vi "_getNbOfElements.vi"(11 "VariantBuffer in":refnum<class "VariantBuffer.lvclass">) -> (2 "nbElements":i32)   [LabVIEW 2013, in "CircularBuffer.lvlib" / "VariantBuffer.lvclass"]
uses:
  VariantBuffer.lvclass
  VariantBuffer.lvclass/VariantBuffer.ctl
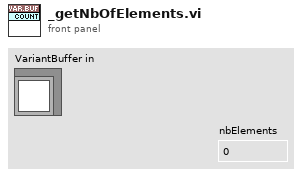
[diagram p1: front panel]
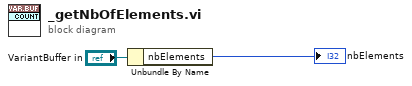
[diagram p0: block diagram]
diagram:
  n1 = Unbundle By Name("VariantBuffer in") -> ("nbElements"=→"nbElements":i32)
